vi "USB6343_initialize(1).vi"() -> (0 "error out":errorcluster caption="错误输出", 3 "tasks":T1)   [LabVIEW 2013]
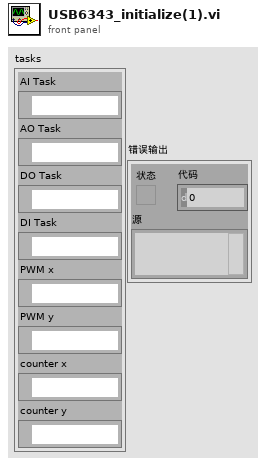
[diagram p1: front panel]
types:
  T1 = cluster{"AI Task":refnum<k21>, "AO Task":refnum<k21>, "DO Task":refnum<k21>, "DI Task":refnum<k21>, "PWM x":refnum<k21>, "PWM y":refnum<k21>, "counter x":refnum<k21>, "counter y":refnum<k21>}
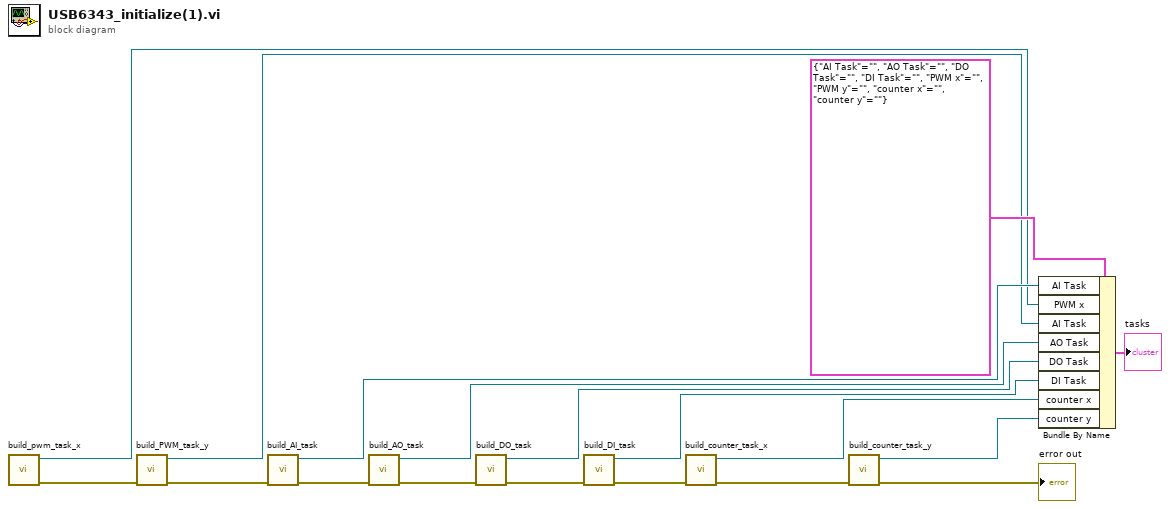
[diagram p0: block diagram]
diagram:
  n1 = call "build_pwm_task_x.vi"() -> ("error out"=w10:errorcluster, "task out"=w8:refnum<k21>)  [unwired: 10 in]
  n2 = call "build_PWM_task_y.vi"("error in"=w10) -> ("error out"=w9:errorcluster, "task out"=w7:refnum<k21>)  [unwired: 9 in]
  n3 = call "build_AI_task.vi"("error in"=w9) -> ("error out"=w15:errorcluster, "task out"=w17:refnum<k21>)  [unwired: 9 in]
  n4 = call "build_AO_task.vi"("error in"=w15) -> ("error out"=w13:errorcluster, "task out"=w16:refnum<k21>)  [unwired: 9 in]
  n5 = call "build_DO_task.vi"("error in"=w13) -> ("error out"=w12:errorcluster, "task out"=w11:refnum<k21>)  [unwired: 9 in]
  n6 = call "build_DI_task.vi"("error in"=w12) -> ("error out"=w6:errorcluster, "task out"=w14:refnum<k21>)  [unwired: 9 in]
  n7 = call "build_counter_task_x.vi"("error in"=w6) -> ("error out"=w5:errorcluster, "task out"=w3:refnum<k21>)  [unwired: 9 in]
  n8 = call "build_counter_task_y.vi"("error in"=w5) -> ("error out"=→"error out":errorcluster, "task out"=w2:refnum<k21>)  [unwired: 9 in]
  n9 = Bundle By Name(cluster=T1 {"AI Task"="", "AO Task"="", "DO Task"="", "DI Task"="", "PWM x"="", "PWM y"="", "counter x"="", "counter y"=""}, "AI Task"=w17, "PWM x"=w8, "AI Task"=w7, "AO Task"=w16, "DO Task"=w11, "DI Task"=w14, "counter x"=w3, "counter y"=w2) -> (→"tasks":T1)
